vi "MainPicMot.vi"() -> ()   [LabVIEW 2010]
uses:
  <vilib>/Instr/_visa.llb/VISA Flush IO Buffer Mask.ctl
  Variable globale 1.vi
  <vilib>/Instr/_visa.llb/VISA Configure Serial Port (Instr).vi
panel:
  out "Byte Start ?":bool
  out "Retour 2":string
  in  "Donnee":i32=138 min=0 max=255
  in  "Numérique":i32=138 min=138 max=139
  in  "stop secu":bool
  in  "STOP":bool
  out "error out":errorcluster caption="sortie d'erreur"
  in  "baud rate (9600)":u32=9600 caption="débit en bauds (9600)"
  in  "Port Com":refnum<visa-resource-name> caption="Nom de ressource VISA"
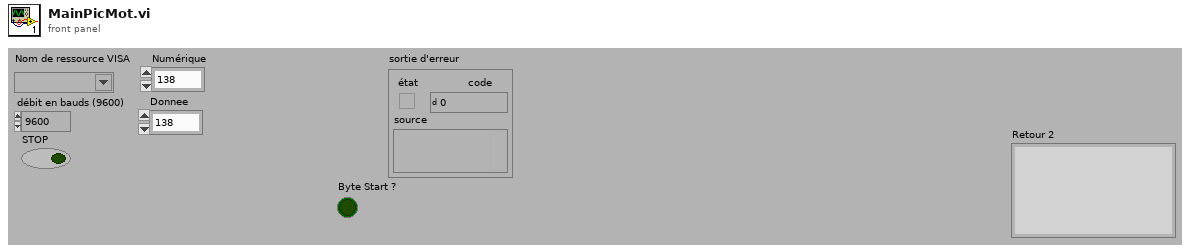
[diagram p1: front panel]
types:
  T1 = typedef "VISA Flush IO Buffer Mask.ctl" = u16
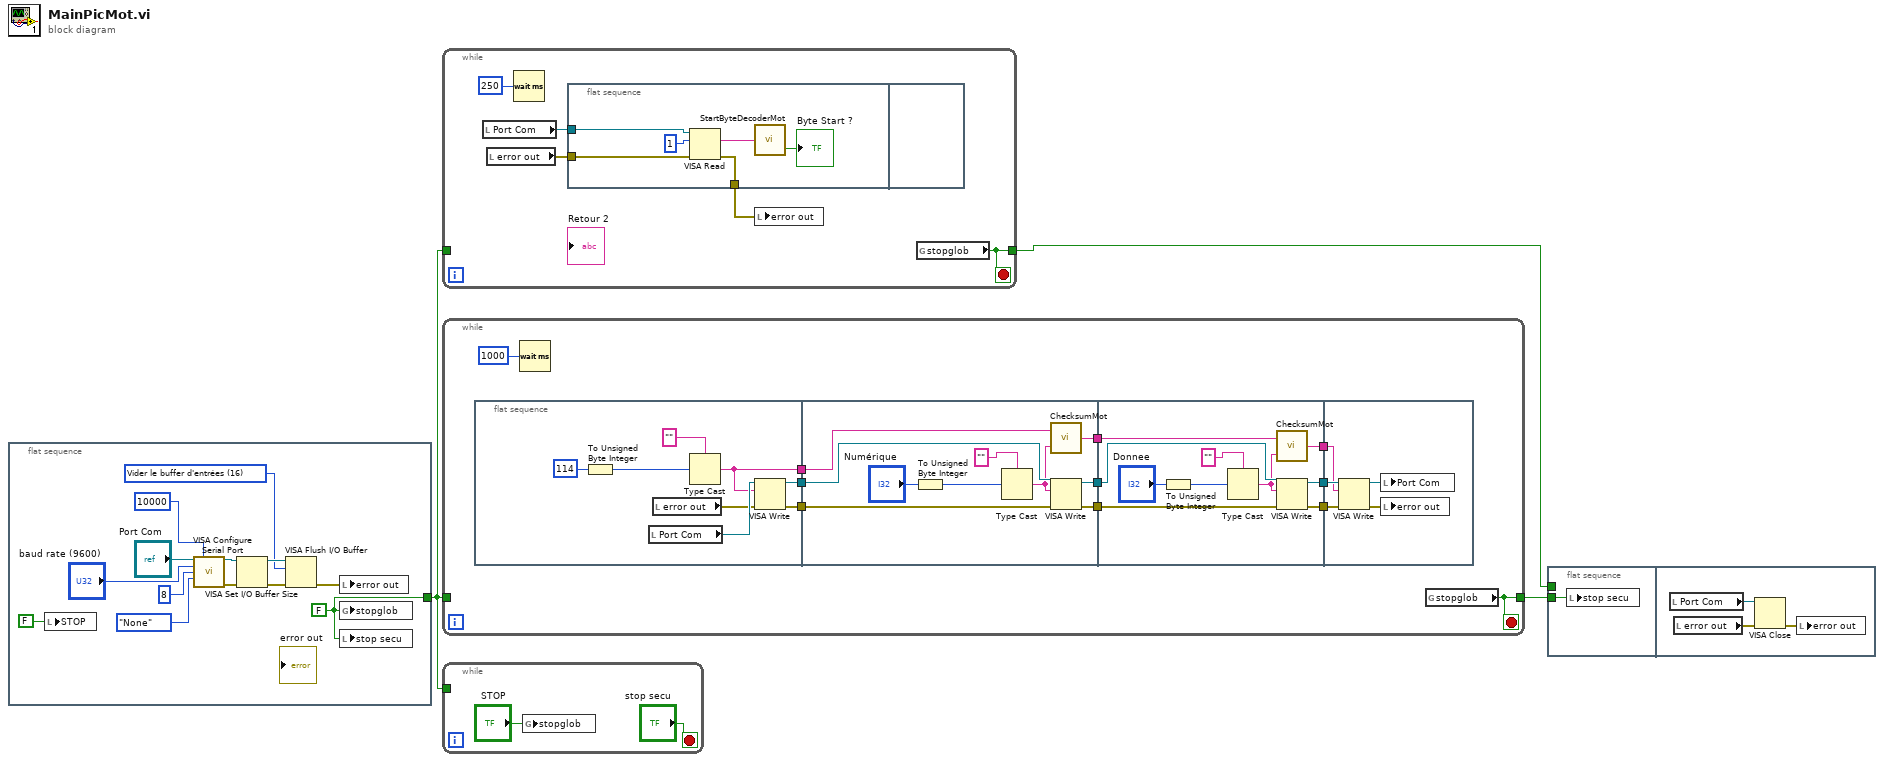
[diagram p0: block diagram]
diagram:
  n1 = flat-sequence {
    tunnel: [w4] -> w2
    frame #0 {
      w4 = FALSE
      w7 = T1 16 items=["Vider le buffer d'entrées"=16, "Écrire le buffer de sorties sur le périphérique"=32, "Vider le buffer d'entrées (Pas d'E/S)"=64, "Vider le buffer de sorties"=128] ("Mask")
      n2 = local write "STOP"(FALSE) -> ()
      n3 = call-poly "VISA Configure Serial Port"("VISA resource name"="Port Com", "timeout (10sec)"=u32 10000, "baud rate (9600)"="baud rate (9600)", "data bits (8)"=u16 8, "parity (0:none)"=enum16{"None", "Odd", "Even", "Mark", "Space"}."None") -> ("VISA resource name out"=w11:refnum<visa-resource-name>, "error out"=w10:errorcluster)  [unwired: 9 in]
      n4 = VISA Set I/O Buffer Size(VISA resource name=w11, error in (no error)=w10) -> (VISA resource name out=w8:refnum<visa-resource-name>, error out=w9:errorcluster)  [unwired: 2 in]
      n5 = VISA Flush I/O Buffer(VISA resource name=w8, mask (16)=w7, error in (no error)=w9) -> (error out=w5:errorcluster)  [unwired: 1 out]
      n6 = local write "error out"(w5) -> ()
      n7 = global write "Variable globale 1.vi" "stopglob"(w4) -> ()
      n8 = local write "stop secu"(w4) -> ()
    }
  }
  n9 = while {
    tunnel: [w21] -> w1
    tunnel: w2 -> [_]
    stop <- w21 stop-if-true
    n10 = local read "Port Com"() -> (w19:refnum<visa-resource-name>)
    n11 = local read "error out"() -> (w18:errorcluster)
    n12 = Wait (ms)(milliseconds to wait=u32 250 ("attente (ms)")) -> ()  [unwired: 1 out]
    n13 = flat-sequence {
      tunnel: w19 -> [w26]
      tunnel: w18 -> [w25]
      tunnel: [w22] -> w17
      frame #0 {
        n14 = VISA Read(VISA resource name=w26, byte count=u32 1 ("nombre d'octets"), error in (no error)=w25) -> (read buffer=w24:string, error out=w22:errorcluster)  [unwired: 2 out]
        n15 = call "StartByteDecoderMot.vi"("byte1"=w24) -> ("Byte Start ?"=→"Byte Start ?":bool)  [unwired: 1 in]
      }
      frame #1 {
      }
    }
    n16 = local write "error out"(w17) -> ()
    n17 = global read "Variable globale 1.vi" "stopglob"() -> (w21:bool)
  }
  n18 = while {
    tunnel: [w28] -> w3
    tunnel: w2 -> [_]
    stop <- w28 stop-if-true
    n19 = flat-sequence {
      tunnel: [w42] -> w38
      tunnel: [w41] -> w37
      tunnel: [w40] -> w32
      tunnel: w38 -> [w54]
      tunnel: w37 -> [w53]
      tunnel: [w52] -> w36
      tunnel: [w51] -> w35
      tunnel: w32 -> [w50]
      tunnel: [w48] -> w31
      tunnel: w36 -> [w66]
      tunnel: w35 -> [w65]
      tunnel: [w62] -> w34
      tunnel: [w61] -> w33
      tunnel: w31 -> [w60]
      tunnel: [w58] -> w30
      tunnel: w34 -> [w71]
      tunnel: w33 -> [w70]
      tunnel: w30 -> [w69]
      frame #0 {
        n20 = To Unsigned Byte Integer(number=114) -> (unsigned 8bit integer=w39:u8)
        n21 = local read "Port Com"() -> (w46:refnum<visa-resource-name>)
        n22 = local read "error out"() -> (w43:errorcluster)
        n23 = Type Cast(type="", x=w39) -> (*(type *) &x=w40:string)
        n24 = VISA Write(VISA resource name=w46, write buffer=w40, error in (no error)=w43) -> (VISA resource name out=w42:refnum<visa-resource-name>, error out=w41:errorcluster)  [unwired: 1 out]
      }
      frame #1 {
        n25 = To Unsigned Byte Integer(number="Numérique") -> (unsigned 8bit integer=w47:u8)
        n26 = Type Cast(type="", x=w47) -> (*(type *) &x=w49:string)
        n27 = call "ChecksumMot.vi"("Byte2"=w49, "Byte1"=w50) -> ("chaîne"=w48:string)
        n28 = VISA Write(VISA resource name=w54, write buffer=w49, error in (no error)=w53) -> (VISA resource name out=w51:refnum<visa-resource-name>, error out=w52:errorcluster)  [unwired: 1 out]
      }
      frame #2 {
        n29 = To Unsigned Byte Integer(number="Donnee") -> (unsigned 8bit integer=w57:u8)
        n30 = Type Cast(type="", x=w57) -> (*(type *) &x=w59:string)
        n31 = call "ChecksumMot.vi"("Byte2"=w59, "Byte1"=w60) -> ("chaîne"=w58:string)
        n32 = VISA Write(VISA resource name=w65, write buffer=w59, error in (no error)=w66) -> (VISA resource name out=w61:refnum<visa-resource-name>, error out=w62:errorcluster)  [unwired: 1 out]
      }
      frame #3 {
        n33 = VISA Write(VISA resource name=w70, write buffer=w69, error in (no error)=w71) -> (VISA resource name out=w68:refnum<visa-resource-name>, error out=w67:errorcluster)  [unwired: 1 out]
        n34 = local write "Port Com"(w68) -> ()
        n35 = local write "error out"(w67) -> ()
      }
    }
    n36 = Wait (ms)(milliseconds to wait=u32 1000 ("attente (ms)")) -> ()  [unwired: 1 out]
    n37 = global read "Variable globale 1.vi" "stopglob"() -> (w28:bool)
  }
  n38 = while {
    tunnel: w2 -> [_]
    stop <- "stop secu" stop-if-true
    n39 = global write "Variable globale 1.vi" "stopglob"("STOP") -> ()
  }
  n40 = flat-sequence {
    tunnel: w3 -> [w74]
    tunnel: w1 -> [_]
    frame #0 {
      n41 = local write "stop secu"(w74) -> ()
    }
    frame #1 {
      n42 = local read "Port Com"() -> (w77:refnum<visa-resource-name>)
      n43 = local read "error out"() -> (w76:errorcluster)
      n44 = VISA Close(VISA resource name=w77, error in (no error)=w76) -> (error out=w75:errorcluster)
      n45 = local write "error out"(w75) -> ()
    }
  }
